vi "AudioTest.Compare Plot to Limit.vi"(8 "error in (no error)":errorcluster, 10 "Plot Limit":T3, 11 "Plot Data":T3) -> (0 "error out":errorcluster, 1 "Result Color":u32(colorbox), 3 "Meas Rslt":T1[](array[typedef]) {"Status" items=["LOG", "PASS", "FAIL", "ERROR"]}, 4 "PASS":bool)   [LabVIEW 2018]
uses:
  TypeDefs/AudioTest.Result Plot Data.ctl
  Common/Utils/Results/Result.Measurement Item.ctl
  Common/Utils/Results/Result.Measurement and Attribute Item Status.ctl
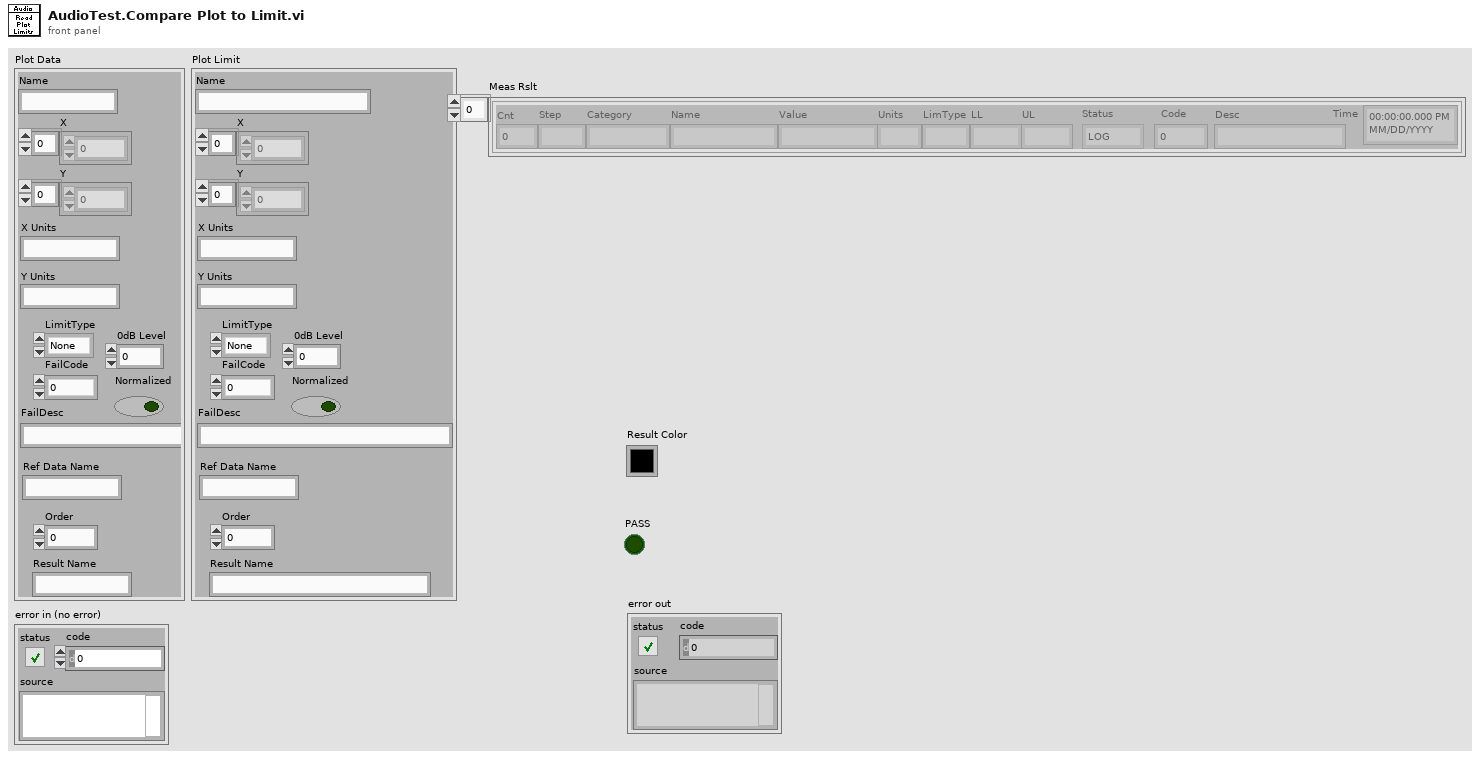
[diagram p1: front panel]
types:
  T1 = typedef "Result.Measurement Item.ctl" = cluster{"Cnt":i32, "Step":string, "Category":string, "Name":string, "Value":string, "Units":string, "LimType":string, "LL":string, "UL":string, "Status":T2, "Code":i32, "Desc":string, "Time":timestamp}
  T2 = typedef "Result.Measurement and Attribute Item Status.ctl" = i32
  T3 = typedef "AudioTest.Result Plot Data.ctl" = cluster{"Order":i32, "Name":string, "X":dbl[], "Y":dbl[], "X Units":string, "Y Units":string, "LimitType":enum16{"None", "LL", "UL"}, "FailCode":i32, "FailDesc":string, "Ref Data Name":string, "Result Name":string, "0dB Level":dbl, "Normalized":bool}
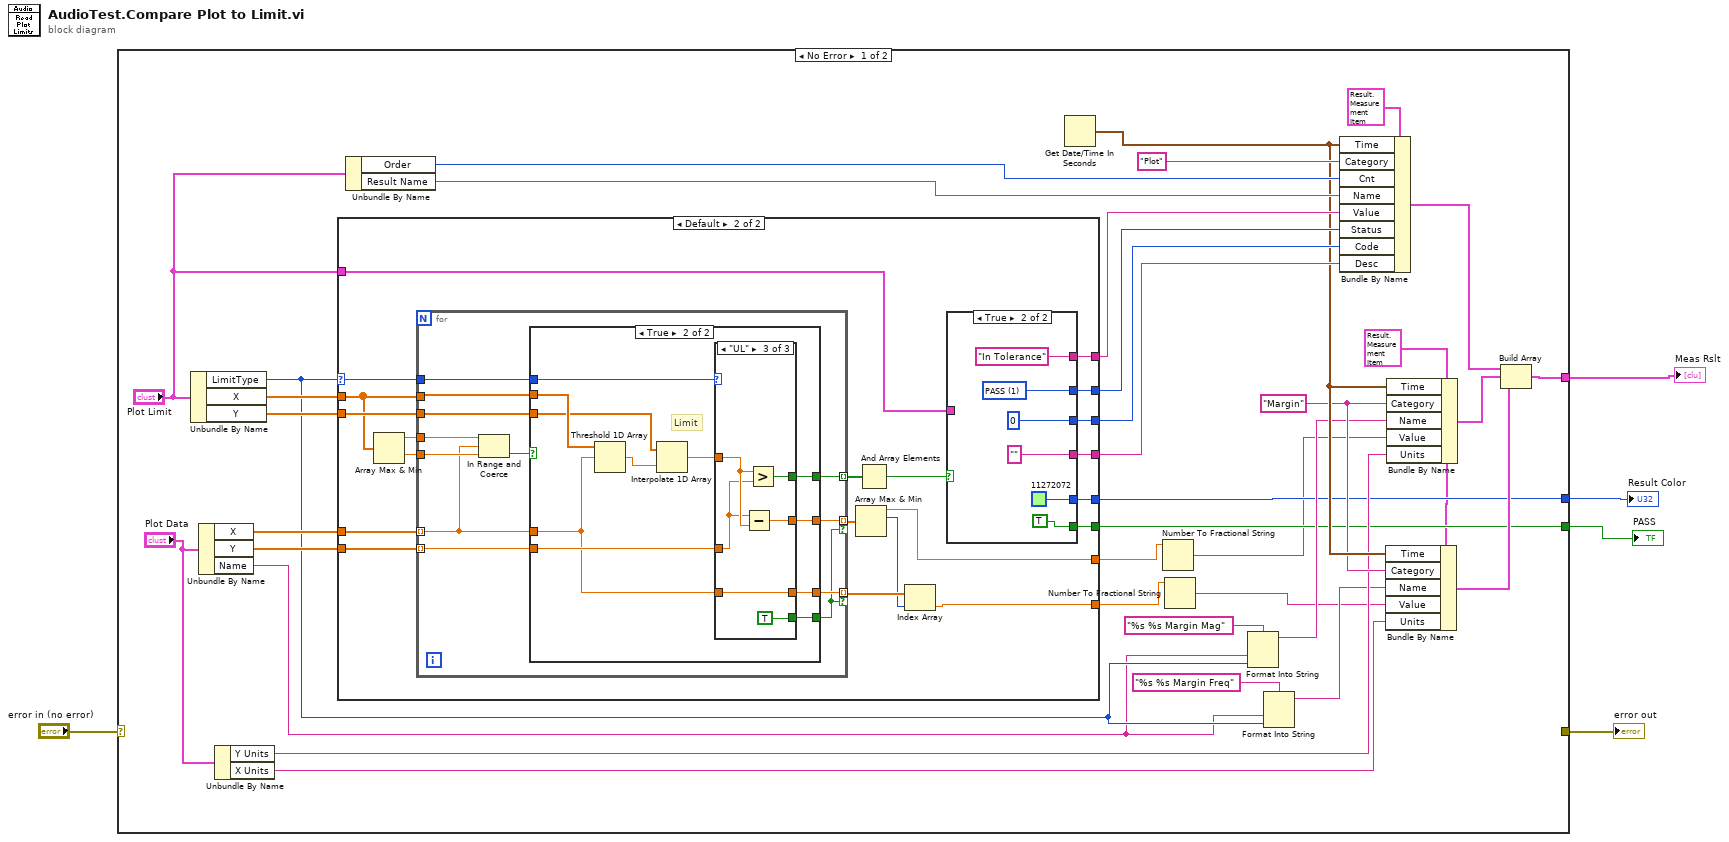
[diagram p0: block diagram]
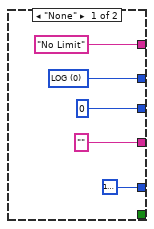
[diagram p2: hidden frame]
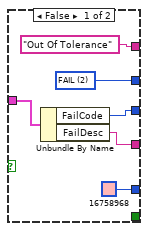
[diagram p3: hidden frame]
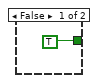
[diagram p4: hidden frame]
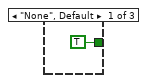
[diagram p5: hidden frame]
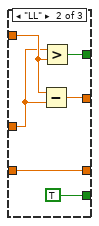
[diagram p6: hidden frame]
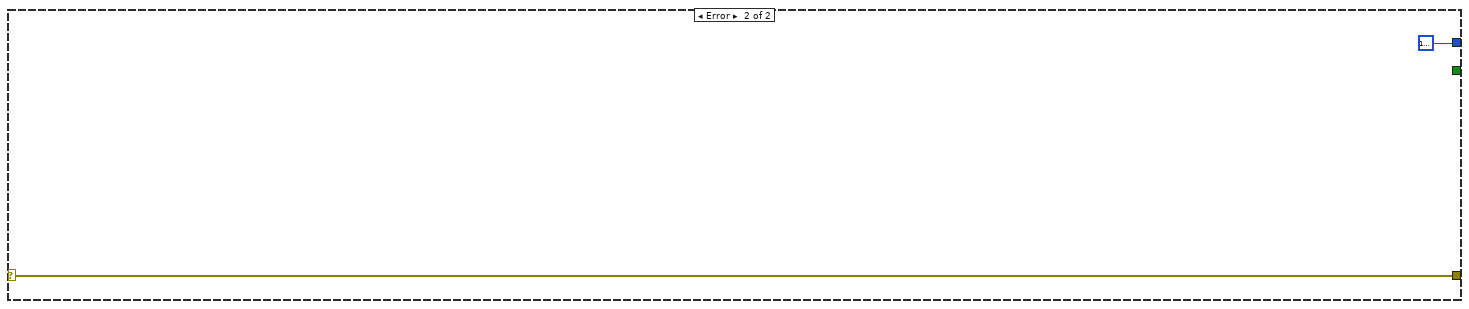
[diagram p7: hidden frame]
diagram:
  n1 = case shown="No Error" "error in (no error)" {
    selector: "error in (no error)" -> [_ w117]
    tunnel: [_ w117] -> w4
    tunnel: [w27 _] -> w1
    tunnel: [w13 u32 16777216] -> w3
    tunnel: [w12 _] -> w2
    frame No Error {
      w10 = T1 {"Cnt"=0, "Step"="", "Category"="", "Name"="", "Value"="", "Units"="", "LimType"="", "LL"="", "UL"="", "Status"=0, "Code"=0, "Desc"="", "Time"=timestamp(0 s since 1904-01-01)} ("Meas")
      w22 = "Margin" ("Category")
      n2 = Unbundle By Name("Plot Limit") -> ("LimitType"=w17:enum16{"None", "LL", "UL"}, "X"=w32:dbl[], "Y"=w31:dbl[])
      n3 = Unbundle By Name("Plot Data") -> ("X"=w29:dbl[], "Y"=w30:dbl[], "Name"=w16:string)
      n4 = Unbundle By Name("Plot Data") -> ("Y Units"=w20:string, "X Units"=w21:string)
      n5 = case shown="Default" w17 {
        selector: w17 -> [_ w60]
        tunnel: w29 -> [_ w66]
        tunnel: w30 -> [_ w65]
        tunnel: w31 -> [_ w64]
        tunnel: w32 -> [_ w61]
        tunnel: "Plot Limit" -> [_ w59]
        tunnel: [w45 w57] -> w36
        tunnel: [0 ("FailCode") w56] -> w35
        tunnel: ["" ("FailDesc") w55] -> w34
        tunnel: ["No Limit" w54] -> w33
        tunnel: [_ w49] -> w8
        tunnel: [_ w48] -> w9
        tunnel: [u32 16777216 w47] -> w13
        tunnel: [_ w46] -> w12
        frame "None" {
          w45 = T2 0 items=["LOG", "PASS", "FAIL", "ERROR"] ("Status")
        }
        frame Default {
          n6 = Array Max & Min(array=w61) -> (max value=w63:dbl, min value=w62:dbl)  [unwired: 2 out]
          n7 = for {
            tunnel: w61 -> [w85]
            tunnel: w64 -> [w84]
            tunnel: w66 -> [w86] mode=indexing
            tunnel: w65 -> [w88] mode=indexing
            tunnel: w63 -> [w90]
            tunnel: w62 -> [w89]
            tunnel: w60 -> [w83]
            tunnel: [w82] -> w53 mode=indexing
            tunnel: [w81] -> w51 mode=indexing if=w79
            tunnel: [w80] -> w52 mode=indexing if=w79
            n8 = In Range and Coerce(upper limit=w90, x=w86, lower limit=w89) -> (In Range?=w87:bool)  [unwired: 1 out]
            n9 = case shown="True" w87 {
              tunnel: w88 -> [_ w98]
              tunnel: w86 -> [_ w95]
              tunnel: w85 -> [_ w102]
              tunnel: w84 -> [_ w100]
              tunnel: w83 -> [_ w99]
              tunnel: [TRUE w97] -> w82
              tunnel: [_ w94] -> w81
              tunnel: [_ w93] -> w80
              tunnel: [_ w92] -> w79
              frame False {
              }
              frame True {
                # "Limit"
                n10 = Threshold 1D Array(2:w95, 3:w102) -> (0:w101:dbl)  [unwired: 1 in]
                n11 = Interpolate 1D Array(1:w101, 2:w100) -> (0:w96:dbl)
                n12 = case shown="\"UL\"" w99 {
                  tunnel: w96 -> [_ w107 w112]
                  tunnel: w98 -> [_ w106 w111]
                  tunnel: [TRUE w109 w115] -> w97
                  tunnel: w95 -> [_ w108 w114]
                  tunnel: [_ w108 w114] -> w94
                  tunnel: [_ w104 w113] -> w93
                  tunnel: [_ TRUE TRUE] -> w92
                  frame "None", Default {
                  }
                  frame "LL" {
                    n13 = Subtract(x=w107, y=w106) -> (x-y=w104:dbl)
                    n14 = Greater?(x=w106, y=w107) -> (0:w109:bool)
                  }
                  frame "UL" {
                    n15 = Subtract(x=w111, y=w112) -> (x-y=w113:dbl)
                    n16 = Greater?(x=w112, y=w111) -> (0:w115:bool)
                  }
                }
              }
            }
          }
          n17 = Array Max & Min(array=w52) -> (max value=w48:dbl, max index (indices)=w50:i32)  [unwired: 2 out]
          n18 = And Array Elements(Boolean array=w53) -> (logical AND=w58:bool)
          n19 = Index Array(array=w51, index=w50) -> (element=w49:dbl)
          n20 = case shown="True" w58 {
            tunnel: w59 -> [w72 _]
            tunnel: [w70 w78] -> w57
            tunnel: [w69 0] -> w56
            tunnel: [w68 ""] -> w55
            tunnel: ["Out Of Tolerance" "In Tolerance"] -> w54
            tunnel: [u32 16758968 u32 11272072] -> w47
            tunnel: [_ TRUE] -> w46
            frame False {
              w70 = T2 2 items=["LOG", "PASS", "FAIL", "ERROR"] ("Status")
              n21 = Unbundle By Name(w72) -> ("FailCode"=w69:i32, "FailDesc"=w68:string)
            }
            frame True {
              w78 = T2 1 items=["LOG", "PASS", "FAIL", "ERROR"] ("Status")
            }
          }
        }
      }
      n22 = Unbundle By Name("Plot Limit") -> ("Order"=w28:i32, "Result Name"=w38:string)
      n23 = Get Date/Time In Seconds() -> (seconds since 1Jan1904=w23:timestamp)
      n24 = Number To Fractional String(number=w9) -> (F-format string=w7:string)  [unwired: 3 in]
      n25 = Number To Fractional String(number=w8) -> (F-format string=w6:string)  [unwired: 3 in]
      n26 = Format Into String(format string="%s %s Margin Mag", w16, w17) -> (resulting string=w15:string)  [unwired: 2 in, 1 out]
      n27 = Format Into String(format string="%s %s Margin Freq", w16, w17) -> (resulting string=w14:string)  [unwired: 2 in, 1 out]
      n28 = Bundle By Name(cluster=T1 {"Cnt"=0, "Step"="", "Category"="", "Name"="", "Value"="", "Units"="", "LimType"="", "LL"="", "UL"="", "Status"=0, "Code"=0, "Desc"="", "Time"=timestamp(0 s since 1904-01-01)} ("Meas"), "Time"=w23, "Category"="Plot", "Cnt"=w28, "Name"=w38, "Value"=w33, "Status"=w36, "Code"=w35, "Desc"=w34) -> (w11:T1)
      n29 = Bundle By Name(cluster=w10, "Time"=w23, "Category"=w22, "Name"=w14, "Value"=w6, "Units"=w21) -> (w24:T1)
      n30 = Bundle By Name(cluster=w10, "Time"=w23, "Category"=w22, "Name"=w15, "Value"=w7, "Units"=w20) -> (w25:T1)
      n31 = Build Array(w11, w25, w24) -> (w27:T1[])
    }
    frame Error {
    }
  }
  "error out" <- w4
  "Meas Rslt" <- w1
  "Result Color" <- w3
  "PASS" <- w2
